vi "Teleop.vi"(10 "Match Info":T1={"Autonomous Elapsed Seconds"=0.0, "TeleOp Elapsed Seconds"=0.0, "Disabled Elapsed Seconds"=0.0, "Visited Autonomous"=FALSE, "Visited TeleOp"=FALSE, "Visited Disabled"=FALSE, "Autonomous Settings"={"Autonomous Style"=enum."Independent", "VI Refnum"=refnum}}, 11 "Call Context":T2) -> ()   [LabVIEW 2011]
doc: "This VI is called for each TeleOp packet received from the DS where the robot is not disabled. It is often used to read from the joysticks and update I/O or to update setpoints for timed control loops. It should complete and return within 20 milliseconds or it may miss DS packets."
uses:
  <vilib>/Rock Robotics/WPI/DriverStation/WPI_DriverStationDerivedRobotMode.ctl
  <vilib>/Rock Robotics/WPI/DriverStation/WPI_DriverStationMatch Info.ctl
  Robot Global Data.vi
panel:
  out "Sonar Voltage":dbl
  out "Direction 2":bool=TRUE
  out "Stopped 2":bool=TRUE
  out "Bottom Rate":dbl
  out "Bottom Distance":dbl
  out "Top Distance":dbl
  out "Top Rate":dbl
  out "Stopped":bool=TRUE
  out "Direction":bool=TRUE
  out "Y Button":bool
  out "X Button":bool
  out "B Button":bool
  out "A Button":bool
  out "Right Analog":bool
  out "Left Analog":bool
  out "Start":bool
  out "RB":bool
  out "LB":bool
  # "Bottom Encoder"
  # "Top Encoder"
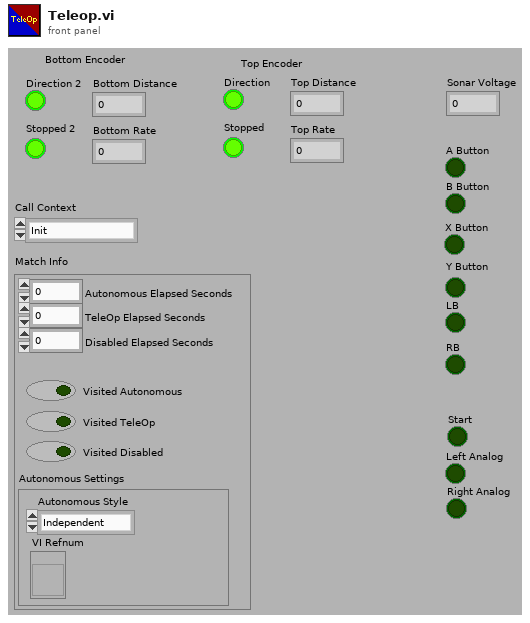
[diagram p1: front panel]
types:
  T1 = typedef "WPI_DriverStationMatch Info.ctl" = cluster{"Autonomous Elapsed Seconds":dbl, "TeleOp Elapsed Seconds":dbl, "Disabled Elapsed Seconds":dbl, "Visited Autonomous":bool, "Visited TeleOp":bool, "Visited Disabled":bool, "Autonomous Settings":cluster{"Autonomous Style":enum16{"Iterative", "Independent"}, "VI Refnum":refnum<vi>}}
  T2 = typedef "WPI_DriverStationDerivedRobotMode.ctl" = enum16{"Init", "Execute", "Stop"}
  T3 = typedef "WPI_JoystickDevRef.ctl" = cluster{"Device":T4}
  T4 = typedef "WPI_JoystickDeviceEnum.ctl" = enum16{"USB 1", "USB 2", "USB 3", "USB 4", "Kinect 1", "Kinect 2"}
  T5 = typedef "WPI_JoystickButtonState.ctl" = cluster{"Button 1":bool, "Button 2":bool, "Button 3":bool, "Button 4":bool, "Button 5":bool, "Button 6":bool, "Button 7":bool, "Button 8":bool, "Button 9":bool, "Button 10":bool, "Button 11":bool, "Button 12":bool}
  T6 = cluster{"axis 1 (x)":dbl, "axis 2 (y)":dbl, "axis 3 (throttle)":dbl, "axis 4":dbl, "axis 5":dbl, "axis 6":dbl}
  T7 = typedef "WPI_EncoderDevRef.ctl" = cluster{"DevStatus":errorcluster, "EncoderIndex":T8, "CounterIndex":T9, "DistancePerCount":dbl, "Decoding Type":T10}
  T8 = typedef "FPGA_EncoderIdx.ctl" = enum8{"Enc 0", "Enc 1", "Enc 2", "Enc 3", "Invalid"}
  T9 = typedef "FPGA_CounterCtrSystemIndex.ctl" = enum8{"Ctr 0", "Ctr 1", "Ctr 2", "Ctr 3", "Ctr 4", "Ctr 5", "Ctr 6", "Ctr 7", "Invalid"}
  T10 = typedef "WPI_EncoderType.ctl" = enum16{"1x", "2x", "4x"}
  T11 = typedef "WPI_AnalogChannelDevRef.ctl" = cluster{"DevStatus":errorcluster, "Analog Module":T12, "Analog Channel":T13}
  T12 = typedef "FPGA_TypedefAnalogModule.ctl" = enum16{"Analog Module 1", "Analog Module 2"}
  T13 = typedef "FPGA_AIChannel.ctl" = enum8{"AI 1", "AI 2", "AI 3", "AI 4", "AI 5", "AI 6", "AI 7", "AI 8", "Invalid"}
  T14 = typedef "WPI_DigitalInputDevRef.ctl" = cluster{"DevStatus":errorcluster, "DIO Channel":T15, "Digital Module":T16}
  T15 = typedef "FPGA_DIOChannel.ctl" = enum8{"DIO 1", "DIO 2", "DIO 3", "DIO 4", "DIO 5", "DIO 6", "DIO 7", "DIO 8", "DIO 9", "DIO 10", "DIO 11", "DIO 12", "DIO 13", "DIO 14", "Invalid"}
  T16 = typedef "FPGA_TypedefDigitalModule.ctl" = enum16{"Digital Module 1", "Digital Module 2"}
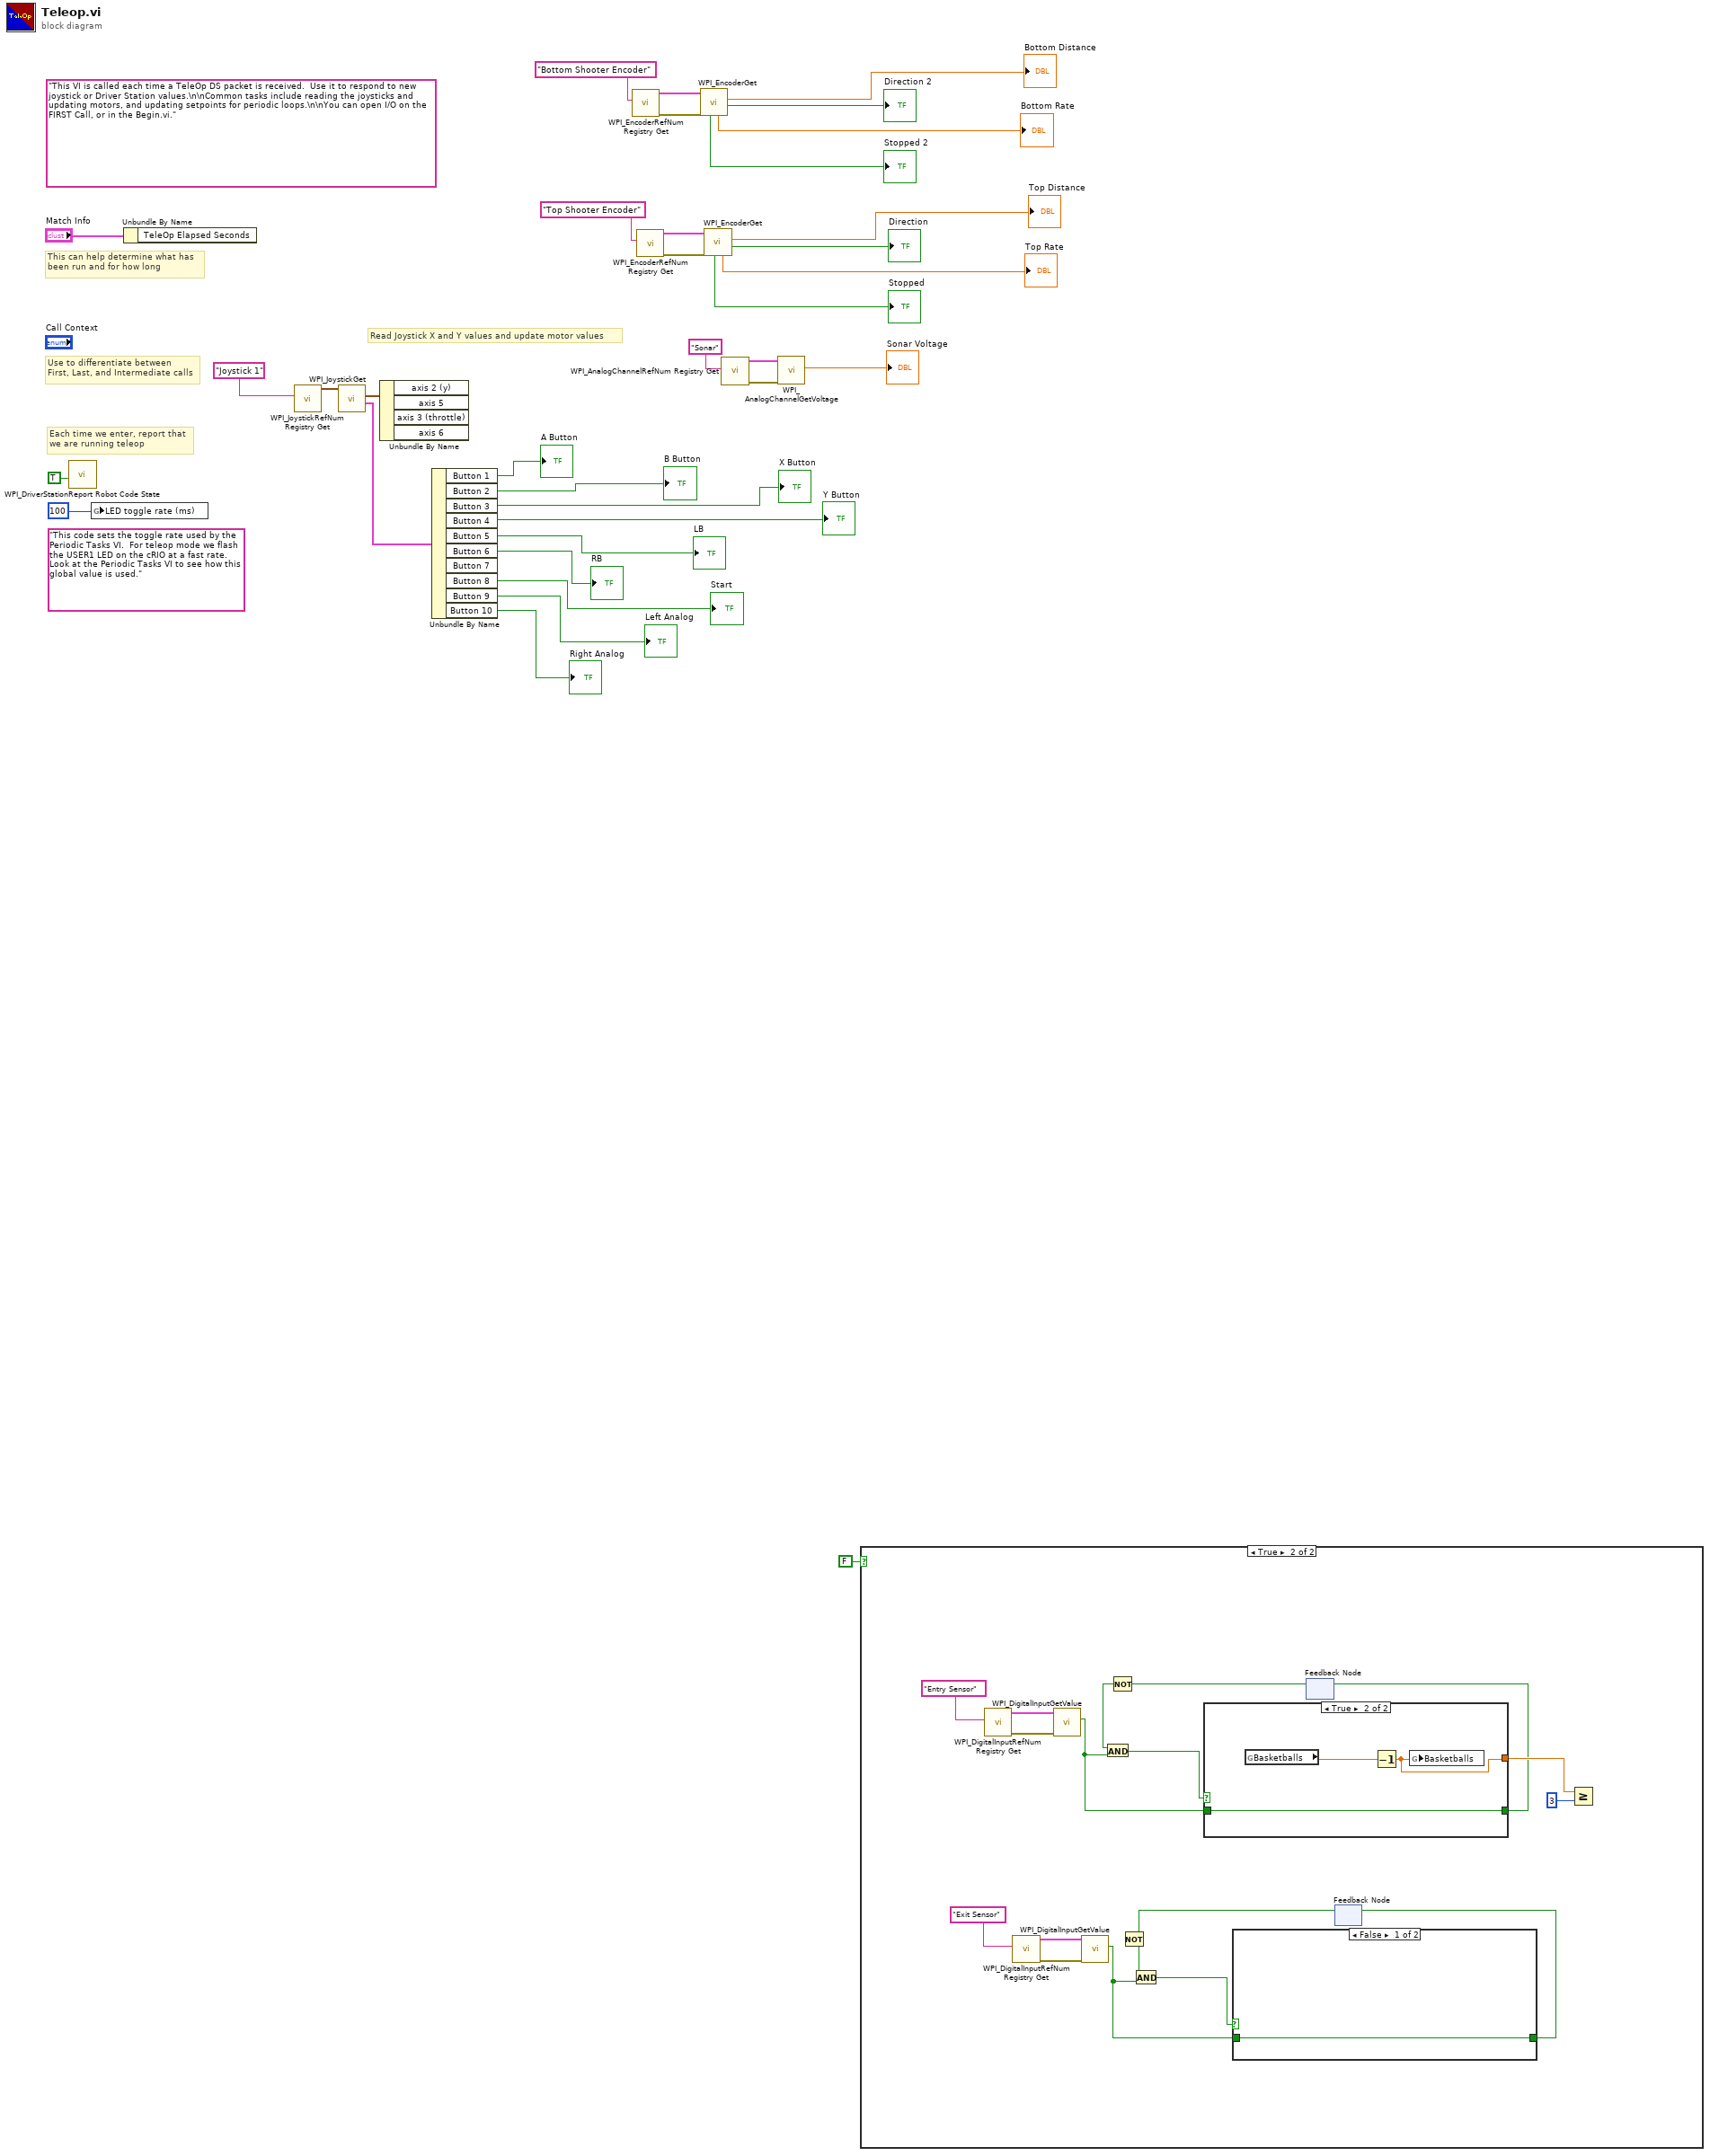
[diagram p0: block diagram]
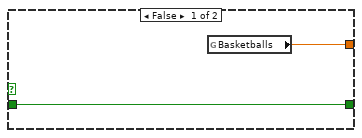
[diagram p3: hidden frame]
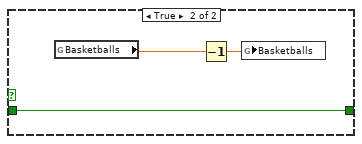
[diagram p4: hidden frame]
diagram:
  (unwired) "This code sets the toggle rate used by the Periodic Tasks VI.  For teleop mode we flash the USER1 LED on the cRIO at a fast rate.  Look at the Periodic Tasks VI to see how this global value is used."
  (unwired) "This VI is called each time a TeleOp DS packet is received.  Use it to respond to new joystick or Driver Station values.\n\nCommon tasks include reading the joysticks and updating motors, and updating setpoints for periodic loops.\n\nYou can open I/O on the FIRST Call, or in the Begin.vi."
  # "Each time we enter, report that\nwe are running teleop"
  # "Use to differentiate between\nFirst, Last, and Intermediate calls"
  # "This can help determine what has\nbeen run and for how long"
  # "Read Joystick X and Y values and update motor values"
  n1 = call <vilib>:"WPI_DriverStationReport Robot Code State.vi"("TeleOp"=TRUE ("Autonomous")) -> ()  [unwired: 10 in, 1 out]
  n2 = global write "Robot Global Data.vi" "LED toggle rate (ms)"(u32 100 ("LED ms toggle rate")) -> ()
  n3 = Unbundle By Name("Match Info") -> ()  [unwired: 1 out]
  n4 = call <vilib>:"WPI_JoystickRefNum Registry Get.vi"("refnum name"="Joystick 1") -> ("JoystickDevRef"=w32:T3)  [unwired: 1 in, 9 out]
  n5 = call <vilib>:"WPI_JoystickGet.vi"("JoystickDevRef"=w32) -> ("Buttons"=w29:T5, "Axes"=w34:T6)  [unwired: 1 in, 4 out]
  n6 = Unbundle By Name(w34) -> ()  [unwired: 4 out]
  n7 = Unbundle By Name(w29) -> ("Button 1"=→"A Button":bool, "Button 2"=→"B Button":bool, "Button 3"=→"X Button":bool, "Button 4"=→"Y Button":bool, "Button 5"=→"LB":bool, "Button 6"=→"RB":bool, "Button 8"=→"Start":bool, "Button 9"=→"Left Analog":bool, "Button 10"=→"Right Analog":bool)  [unwired: 1 out]
  n8 = call <vilib>:"WPI_EncoderRefNum Registry Get.vi"("refnum name"="Bottom Shooter Encoder") -> ("error out"=w1:errorcluster, "EncoderDevRef"=w7:T7)  [unwired: 9 in]
  n9 = call <vilib>:"WPI_EncoderRefNum Registry Get.vi"("refnum name"="Top Shooter Encoder") -> ("error out"=w2:errorcluster, "EncoderDevRef"=w18:T7)  [unwired: 9 in]
  n10 = call <vilib>:"WPI_EncoderGet.vi"("error in (no error)"=w1, "EncoderDevRef"=w7) -> ("Direction"=→"Direction 2":bool, "Distance"=→"Bottom Distance":dbl, "Rate"=→"Bottom Rate":dbl, "Stopped"=→"Stopped 2":bool)  [unwired: 4 in, 2 out]
  n11 = call <vilib>:"WPI_EncoderGet.vi"("error in (no error)"=w2, "EncoderDevRef"=w18) -> ("Direction"=→"Direction":bool, "Distance"=→"Top Distance":dbl, "Rate"=→"Top Rate":dbl, "Stopped"=→"Stopped":bool)  [unwired: 4 in, 2 out]
  n12 = call <vilib>:"WPI_AnalogChannelRefNum Registry Get.vi"("refnum name"="Sonar") -> ("error out"=w5:errorcluster, "AIDeviceRef"=w6:T11)  [unwired: 9 in]
  n13 = call <vilib>:"WPI_AnalogChannelGetVoltage.vi"("error in (no error)"=w5, "AIDeviceRef"=w6) -> ("Voltage"=→"Sonar Voltage":dbl)  [unwired: 7 in, 2 out]
  n14 = case shown="True" FALSE {
    frame False {
    }
    frame True {
      n15 = call <vilib>:"WPI_DigitalInputRefNum Registry Get.vi"("refnum name"="Entry Sensor") -> ("error out"=w41:errorcluster, "DigitalInputDevRef"=w42:T14)  [unwired: 9 in]
      n16 = call <vilib>:"WPI_DigitalInputRefNum Registry Get.vi"("refnum name"="Exit Sensor") -> ("error out"=w49:errorcluster, "DigitalInputDevRef"=w50:T14)  [unwired: 9 in]
      n17 = call <vilib>:"WPI_DigitalInputGetValue.vi"("error in (no error)"=w41, "DigitalInputDevRef"=w42) -> ("Value"=w37:bool)  [unwired: 7 in, 2 out]
      n18 = call <vilib>:"WPI_DigitalInputGetValue.vi"("error in (no error)"=w49, "DigitalInputDevRef"=w50) -> ("Value"=w45:bool)  [unwired: 7 in, 2 out]
      n19 = feedback #1() -> (w39:bool)  [unwired: 1 in]
      n20 = Not(x=w39) -> (.not. x?=w38:bool)
      n21 = And(x=w38, y=w37) -> (x .and. y?=w40:bool)
      n22 = case shown="True" w40 {
        tunnel: [w55 w58] -> w36
        tunnel: w37 -> [w55 w58]
        tunnel: [w54 w56] -> w53
        frame False {
          n23 = global read "Robot Global Data.vi" "Basketballs"() -> (w54:dbl)
        }
        frame True {
          n24 = global read "Robot Global Data.vi" "Basketballs"() -> (w57:dbl)
          n25 = Decrement(x=w57) -> (x-1=w56:dbl)
          n26 = global write "Robot Global Data.vi" "Basketballs"(w56) -> ()
        }
      }
      n27 = feedback-in #1(w36) -> ()
      n28 = feedback #2() -> (w46:bool)  [unwired: 1 in]
      n29 = Not(x=w46) -> (.not. x?=w44:bool)
      n30 = And(x=w44, y=w45) -> (x .and. y?=w48:bool)
      n31 = case shown="False" w48 {
        tunnel: [w59 w62] -> w47
        tunnel: w45 -> [w59 w62]
        frame False {
        }
        frame True {
          n32 = global read "Robot Global Data.vi" "Basketballs"() -> (w61:dbl)
          n33 = Decrement(x=w61) -> (x-1=w60:dbl)
          n34 = global write "Robot Global Data.vi" "Basketballs"(w60) -> ()
        }
      }
      n35 = feedback-in #2(w47) -> ()
      n36 = Greater Or Equal?(x=w53, y=3) -> ()  [unwired: 1 out]
    }
  }
